vi "WPI_CameraSend Images To PC LoopCustom.vi"(8 "error in (no error)":errorcluster, 11 "CameraDevRef":T1) -> ()   [LabVIEW 2015]
doc: "This VI is used to send images to the dashboard using the second enet port on the 8 slot controller. This is provided for compatibility, but is higher overhead than using the Camera MJPG approach.\n\nThis software is licensed. Open the labview\\readme\\WPI Robotics Library Open Source License.txt file for more information."
uses:
  <vilib>/Rock Robotics/WPI/Camera/WPI_CameraDevRef.ctl
  <vilib>/Rock Robotics/SystemInterfaces/NetworkCommunication/NetComm_UsageReport_ResourceType.ctl
  Robot Global Data.vi
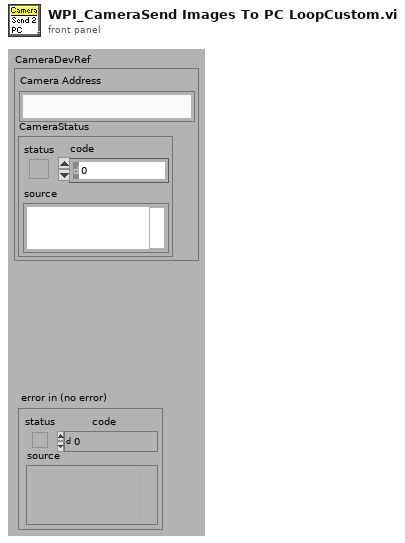
[diagram p1: front panel]
types:
  T1 = typedef "WPI_CameraDevRef.ctl" = cluster{"Camera Address":string, "CameraStatus":errorcluster}
  T2 = cluster{"fps":i32, "compression":i32, "compression 2":i32}
  T3 = typedef "NetComm_UsageReport_ResourceType.ctl" = enum8{"Controller", "Module", "Language", "CANPlugin", "Accelerometer", "ADXL345", "AnalogChannel", "AnalogTrigger", "AnalogTriggerOutput", "CANJaguar", "Compressor", "Counter", "Dashboard", "DigitalInput", "DigitalOutput", "DriverStationCIO", "DriverStationEIO", "DriverStationLCD", "Encoder", "GearTooth", "Gyro", "I2C", "Framework", "Jaguar", "Joystick", "Kinect", "KinectStick", "PIDController", "Preferences", "PWM", "Relay", "RobotDrive", "SerialPort", "Servo", "Solenoid", "SPI", "Task", "Ultrasonic", "Victor", "Button", "Command", "AxisCamera", "PCVideoServer", "SmartDashboard", "Talon", "HiTechnicColorSensor", "HiTechnicAccel", "HiTechnicCompass", "SRF08", "AnalogOutput", "Victor SP", "Talon SRX", "CAN Talon SRX", "ADXL362 Accel", "ADXRS450 Gyro", "Rev SPARK", "Mindsensors SD540", "Digital Filter"}
  T4 = enum16{"Update Mode", "Get Image", "Get Image Data"}
  T5 = typedef "Image Type" = u32
  T6 = typedef "IMAQ Image.ctl" = refnum<image>
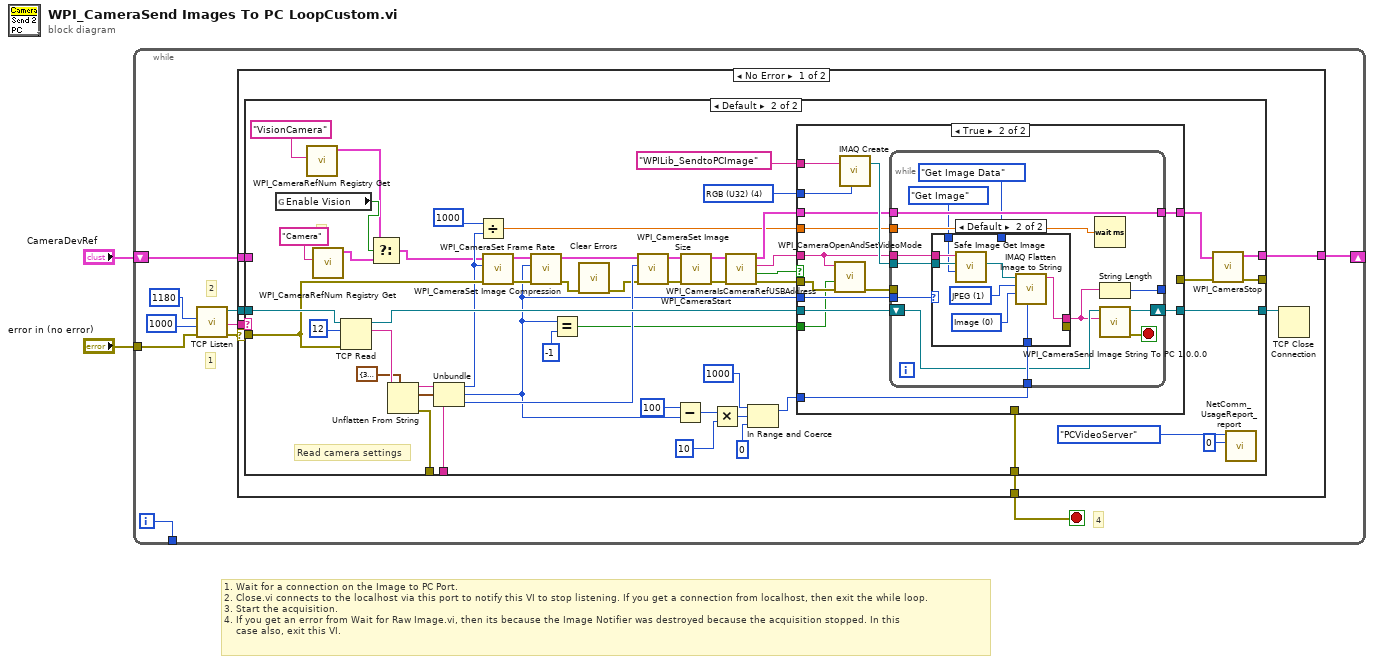
[diagram p0: block diagram]
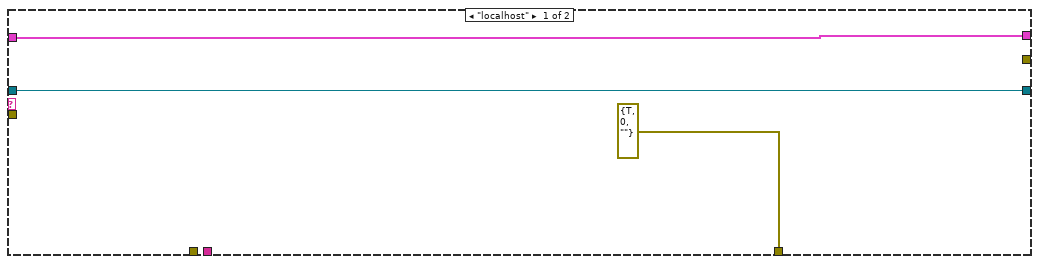
[diagram p2: hidden frame]
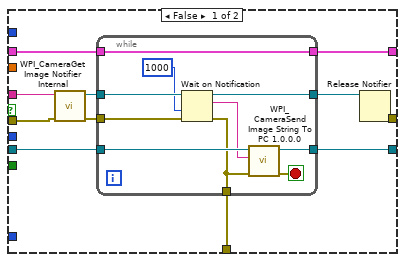
[diagram p3: hidden frame]
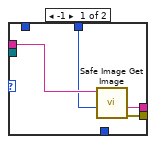
[diagram p4: hidden frame]
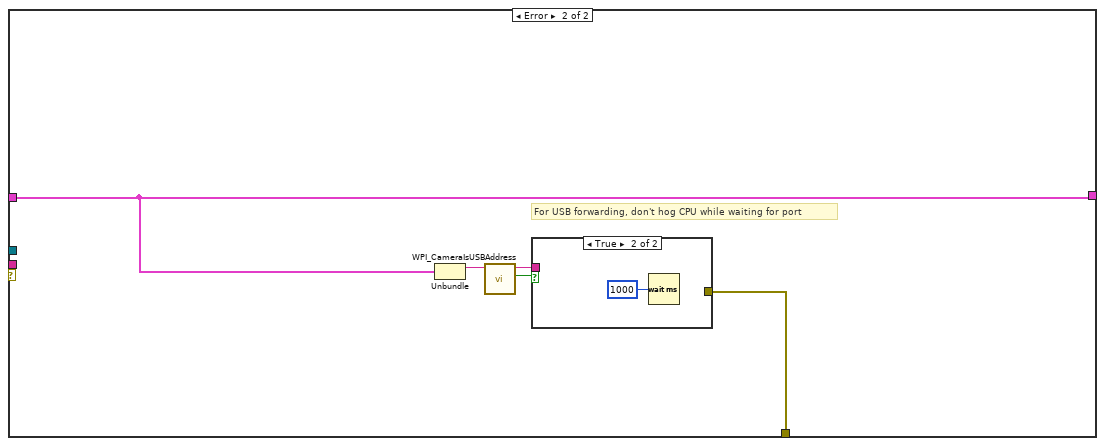
[diagram p5: hidden frame]
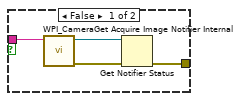
[diagram p6: hidden frame]
diagram:
  # "1. Wait for a connection on the Image to PC Port.\n2. Close.vi connects to the localhost via this port to notify this VI to stop listening. If you get a connection from localhost, then exit the while loop.\n3. Start the acquisition.\n4. If you get an error from Wait for Raw Image.vi, then its because the Image Notifier was destroyed because the acquisition stopped. In this\n    case also, exit this VI."
  n1 = while {
    tunnel: "error in (no error)" -> [w9]
    shift-right: [w12] -> _
    shift-left: "CameraDevRef" -> [w10]
    tunnel: [w3] -> _
    i -> [w3]
    stop <- w7 stop-if-true
    # "4"
    # "1"
    # "2"
    n2 = call <vilib>:"TCP Listen.vi"("error in (no error)"=w9, "timeout ms (wait forever: -1)"=u16 1000 ("port"), "port"=u16 1180) -> ("error out"=w5:errorcluster, "remote address"=w11:string, "connection ID"=w8:refnum<k5>)  [unwired: 1 in, 5 out]
    n3 = case shown="No Error" w5 {
      selector: w5 -> [w13 _]
      tunnel: [w19 w138] -> w12
      tunnel: w11 -> [w18 _]
      tunnel: w10 -> [w17 w138]
      tunnel: w8 -> [w16 _]
      tunnel: [w15 w139] -> w7
      frame No Error {
        n4 = case shown="Default" w18 {
          tunnel: [w22 w72] -> w19
          tunnel: w17 -> [w22 _]
          tunnel: w13 -> [_ w51]
          tunnel: w16 -> [w20 w58]
          tunnel: [errorcluster {"status"=TRUE, "code"=0, "source"=""} ("error out 2") w74] -> w15
          tunnel: [w20 w73] -> w14
          tunnel: [_ w71] -> _
          tunnel: [_ w30] -> _
          tunnel: [_ w29] -> _
          frame "localhost" {
          }
          frame Default {
            w65 = T5 4 items=["Grayscale (U8)", "Grayscale (I16)", "Grayscale (SGL)", "Complex (CSG)", "RGB (U32)", "HSL (U32)", "RGB (U64)", "Grayscale (U16)"] ("Image Type")
            # "Read camera settings"
            # "3"
            n5 = global read "Robot Global Data.vi" "Enable Vision"() -> (w27:bool)
            n6 = call <vilib>:"WPI_CameraRefNum Registry Get.vi"("refnum name"="VisionCamera") -> ("CameraDevRef"=w26:T1)  [unwired: 9 in, 1 out]
            n7 = call <vilib>:"WPI_CameraRefNum Registry Get.vi"("refnum name"="Camera") -> ("CameraDevRef"=w25:T1)  [unwired: 9 in, 1 out]
            n8 = TCP Read(connection ID=w58, bytes to read=12, error in (no error)=w51) -> (connection ID out=w57:refnum<k5>, data out=w55:string)  [unwired: 2 in, 1 out]
            n9 = Select(t=w26, s=w27, f=w25) -> (s? t:f=w28:T1)
            n10 = Unflatten From String(type=T2 {"fps"=30, "compression"=32, "compression 2"=32} ("Camera Settings"), binary string=w55) -> (rest of the binary string=w29:string, value=w48:T2, error out=w30:errorcluster)  [unwired: 3 in]
            n11 = Unbundle(w48) -> ("fps"=w45:i32, "compression"=w34:i32, "compression 2"=w47:i32)
            n12 = Divide(x=u16 1000 ("port"), y=w45) -> (x/y=w44:dbl)
            n13 = call <vilib>:"WPI_CameraSet Frame Rate.vi"("error in (no error)"=w51, "Frame Rate (fps)"=w45, "CameraDevRef"=w28) -> ("error out"=w50:errorcluster, "CameraDevRef Out"=w54:T1)  [unwired: 7 in]
            n14 = call <vilib>:"WPI_CameraSet Image Compression.vi"("error in (no error)"=w50, "Compression"=w34, "CameraDevRef"=w54) -> ("error out"=w32:errorcluster, "CameraDevRef Out"=w53:T1)  [unwired: 7 in]
            n15 = Equal?(x=w34, y=-1) -> (x = y?=w33:bool)
            n16 = call <vilib>:"Clear Errors.vi"("error in (no error)"=w32) -> ("error out"=w31:errorcluster)  [unwired: 5 in, 1 out]
            n17 = call <vilib>:"WPI_CameraSet Image Size.vi"("error in (no error)"=w31, "Image Size"=w47, "CameraDevRef"=w53) -> ("error out"=w49:errorcluster, "CameraDevRef Out"=w52:T1)  [unwired: 7 in]
            n18 = Subtract(x=100, y=w34) -> (x-y=w39:i32)
            n19 = call <vilib>:"WPI_CameraStart.vi"("error in (no error)"=w49, "CameraDevRef"=w52) -> ("error out"=w62:errorcluster, "CameraDevRef"=w60:T1)  [unwired: 8 out]
            n20 = Multiply(x=w39, y=10) -> (x*y=w41:i32)
            n21 = call <vilib>:"WPI_CameraIsCameraRefUSBAddress.vi"("error in (no error)"=w62, "CameraDevRef"=w60) -> ("error out"=w61:errorcluster, "USB?"=w63:bool, "Camera Address Out"=w64:string, "CameraDevRef out"=w59:T1)  [unwired: 6 in]
            n22 = In Range and Coerce(upper limit=1000, x=w41, lower limit=0) -> (coerced(x)=w37:i32)  [unwired: 1 out]
            n23 = case shown="True" w63 {
              tunnel: w57 -> [w85 w109]
              tunnel: [w84 _] -> w74
              tunnel: [w83 w108] -> w73
              tunnel: w61 -> [w82 w99]
              tunnel: w64 -> [w80 w98]
              tunnel: [w79 w103] -> w70
              tunnel: w59 -> [w78 w104]
              tunnel: [w76 _] -> w69
              tunnel: "WPILib_SendtoPCImage" -> [_ w106]
              tunnel: w65 -> [_ w105]
              tunnel: w37 -> [_ w102]
              tunnel: w44 -> [_ w101]
              tunnel: w34 -> [_ w100]
              tunnel: w33 -> [_ w96]
              frame False {
                n24 = call <vilib>:"WPI_CameraGet Image Notifier Internal.vi"("error in (no error)"=w82, "Camera Address"=w80) -> ("error out"=w81:errorcluster, "Image Notifier"=w77:refnum<notifier>)  [unwired: 8 out]
                n25 = while {
                  tunnel: w81 -> [w91]
                  tunnel: w85 -> [w95]
                  tunnel: [w88] -> w84
                  tunnel: [w93] -> w83
                  tunnel: [w92] -> w79
                  tunnel: w78 -> [w92]
                  tunnel: w77 -> [w90]
                  tunnel: [w86] -> w75
                  stop <- w94 stop-if-true
                  n26 = Wait on Notification(notifier=w90, timeout in ms (-1)=1000 ("Timeout in ms (-1)"), error in (no error)=w91) -> (notifier out=w86:refnum<notifier>, notification=w89:string, error out=w88:errorcluster)  [unwired: 2 out]
                  n27 = call <vilib>:"WPI_CameraSend Image String To PC 1.0.0.0.vi"("error in (no error)"=w88, "String"=w89, "TCP Connection ID"=w95) -> ("error out"=w94:errorcluster, "TCP Connection ID out"=w93:refnum<k5>)  [unwired: 7 out]
                }
                n28 = Release Notifier(notifier=w75) -> (error out=w76:errorcluster)  [unwired: 1 in, 3 out]
              }
              frame True {
                n29 = call <vilib>:"WPI_CameraOpenAndSetVideoMode.vi"("error in (no error)"=w99, "USB JPEG"=w96, "Camera Address Out"=w98) -> ("error out"=w97:errorcluster)  [unwired: 8 in]
                n30 = call "IMAQ Create"("Image Name"=w106, "Image Type"=w105) -> ("New Image"=w107:T6)  [unwired: 3 in, 1 out]
                n31 = while {
                  tunnel: w98 -> [w121]
                  shift-right: [w122] -> w108
                  shift-left: w109 -> [w115]
                  tunnel: w107 -> [w120]
                  tunnel: [w118] -> w103
                  tunnel: w104 -> [w118]
                  tunnel: w102 -> [w117]
                  tunnel: w101 -> [w116]
                  tunnel: [w113] -> _
                  tunnel: w100 -> [w112]
                  tunnel: w97 -> [_]
                  stop <- w119 stop-if-true
                  n32 = case shown="Default" w112 {
                    tunnel: [w125 w134] -> w114
                    tunnel: w121 -> [w126 w130]
                    tunnel: w120 -> [_ w129]
                    tunnel: w117 -> [_ w131]
                    tunnel: [w124 _] -> _
                    tunnel: T4."Get Image Data" ("Operation") -> [w123 _]
                    tunnel: T4."Get Image" ("Operation") -> [_ w127]
                    frame -1 {
                      n33 = call <vilib>:"Safe Image Get Image.vi"("Operation"=w123, "Session In"=w126) -> ("error out"=w124:errorcluster, "Image Data String"=w125:string)  [unwired: 6 in, 2 out]
                    }
                    frame Default {
                      w132 = 0 items=["Image", "Image and Vision Info", "Reference to Image"] ("Type of Flatten (Image and Vision Info)")
                      w133 = 1 items=["None", "JPEG", "PACKED BINARY"] ("Compression (None)")
                      n34 = call <vilib>:"Safe Image Get Image.vi"("Operation"=w127, "Image In"=w129, "Session In"=w130) -> ("Image Out"=w128:T6)  [unwired: 5 in, 3 out]
                      n35 = call "IMAQ Flatten Image to String"("Quality (750)"=w131, "Type of Flatten (Image and Vision Info)"=w132, "Compression (None)"=w133, "Image"=w128) -> ("Data String"=w134:string)  [unwired: 6 in, 1 out]
                    }
                  }
                  n36 = Wait (ms)(milliseconds to wait=w116) -> ()  [unwired: 1 out]
                  n37 = String Length(string=w114) -> (length=w113:i32)
                  n38 = call <vilib>:"WPI_CameraSend Image String To PC 1.0.0.0.vi"("String"=w114, "TCP Connection ID"=w115) -> ("error out"=w119:errorcluster, "TCP Connection ID out"=w122:refnum<k5>)  [unwired: 1 in, 7 out]
                }
              }
            }
            n39 = call <vilib>:"WPI_CameraStop.vi"("error in (no error)"=w69, "CameraDevRef"=w70) -> ("error out"=w71:errorcluster, "CameraDevRef"=w72:T1)  [unwired: 8 out]
            n40 = call <vilib>:"NetComm_UsageReport_report.vi"("Instance Number"=u8 0, "Resource Type"=NetComm_UsageReport_ResourceType."PCVideoServer") -> ()  [unwired: 10 in]
          }
        }
        n41 = TCP Close Connection(connection ID=w14) -> ()  [unwired: 1 in, 3 out]
      }
      frame Error {
        # "For USB forwarding, don't hog CPU while waiting for port"
        n42 = Unbundle(w138) -> ("Camera Address"=w137:string)  [unwired: 1 out]
        n43 = call <vilib>:"WPI_CameraIsUSBAddress.vi"("Camera Address In"=w137) -> ("USB?"=w135:bool, "Camera Address Out"=w136:string)  [unwired: 8 in, 1 out]
        n44 = case shown="True" w135 {
          tunnel: [w143 _] -> w139
          tunnel: w136 -> [w140 _]
          frame False {
            n45 = call <vilib>:"WPI_CameraGet Acquire Image Notifier Internal.vi"("Camera Address"=w140) -> ("error out"=w141:errorcluster, "Acquire Image Notifier"=w142:refnum<notifier>)  [unwired: 1 in, 8 out]
            n46 = Get Notifier Status(notifier=w142, error in (no error)=w141) -> (error out=w143:errorcluster)  [unwired: 4 out]
          }
          frame True {
            n47 = Wait (ms)(milliseconds to wait=u32 1000) -> ()  [unwired: 1 out]
          }
        }
      }
    }
  }
